vi "F_r_2_vi.vi"() -> ()   [LabVIEW 2018]
uses:
  F_r_var_glob.vi
panel:
  in  "stop":bool
  in  "Numeric 4":dbl
  in  "Numeric 3":dbl
  in  "Numeric 2":dbl
  in  "Numeric":dbl
  # "Durée des phases en secondes"
  # "Phase: 1"
  # "Phase: 2"
  # "Phase: 3"
  # "Phase: 4"
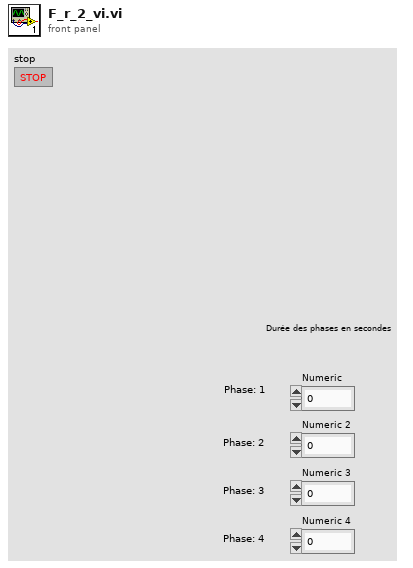
[diagram p1: front panel]
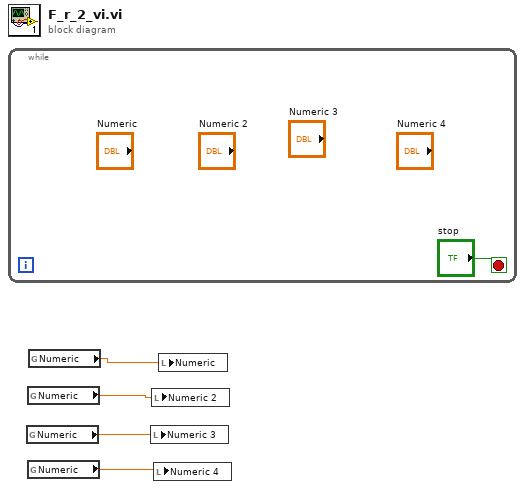
[diagram p0: block diagram]
diagram:
  n1 = while {
    stop <- "stop" stop-if-true
  }
  n2 = global read "F_r_var_glob.vi" "Numeric"() -> (w3:dbl)
  n3 = global read "F_r_var_glob.vi" "Numeric"() -> (w2:dbl)
  n4 = global read "F_r_var_glob.vi" "Numeric"() -> (w4:dbl)
  n5 = global read "F_r_var_glob.vi" "Numeric"() -> (w1:dbl)
  n6 = local write "Numeric 3"(w3) -> ()
  n7 = local write "Numeric 2"(w2) -> ()
  n8 = local write "Numeric 4"(w4) -> ()
  n9 = local write "Numeric"(w1) -> ()
